vi "LangmuirProbeControlV2.vi"() -> ()   [LabVIEW 2014]
uses:
  <vilib>/express/express shared/transition.llb/Dynamic To Waveform Array.vi
  <vilib>/express/express arith-compare/Formula/Block/exnFormulaBlock how many pts in the wave.vi
  <vilib>/express/express shared/ex_Modify Signal Name.vi
  <vilib>/express/express shared/transition.llb/Waveform Array To Dynamic.vi
  <vilib>/express/express arith-compare/Formula/XNode/ExpressFormulaBlockNode.xnode
panel:
  in  "Min Voltage":dbl caption="Amplitude"
  in  "Max Voltage":dbl caption="Amplitude"
  in  "Log Data":bool
  out "I-V Curve":cluster{"Y":dbl[], "Y":dbl[]}[](graph)
  out "Waveform Graph":dynamicdata(graph)
  out "Resistor Voltage In":dbl
  out "Current Measure (V)":dynamicdata(graph) caption="data"
  out "Generated Signal":dynamicdata(graph) caption="Sine"
  in  "stop (F)":bool caption="STOP (F)"
  # "Desired Voltage Swing"
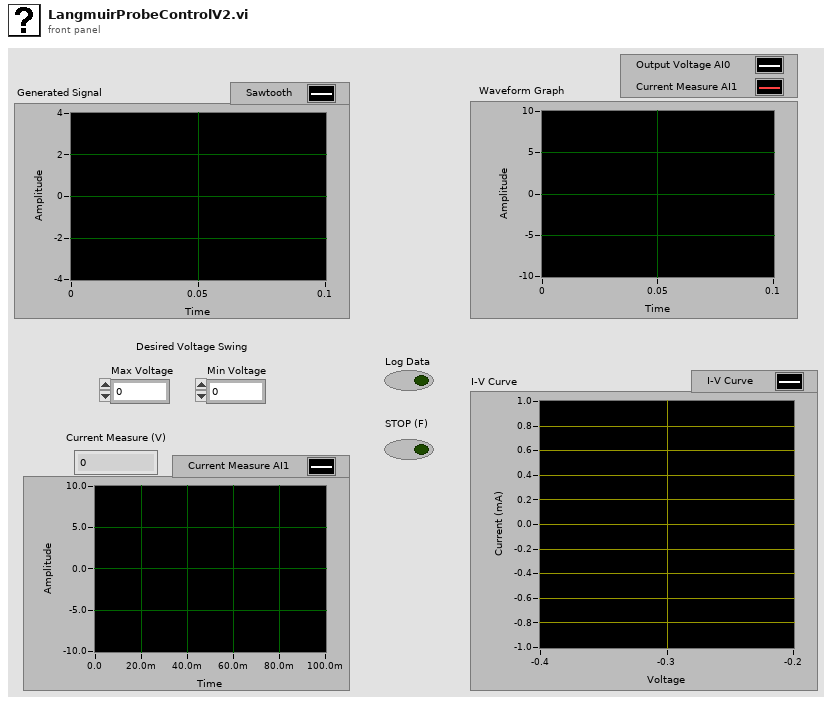
[diagram p1: front panel]
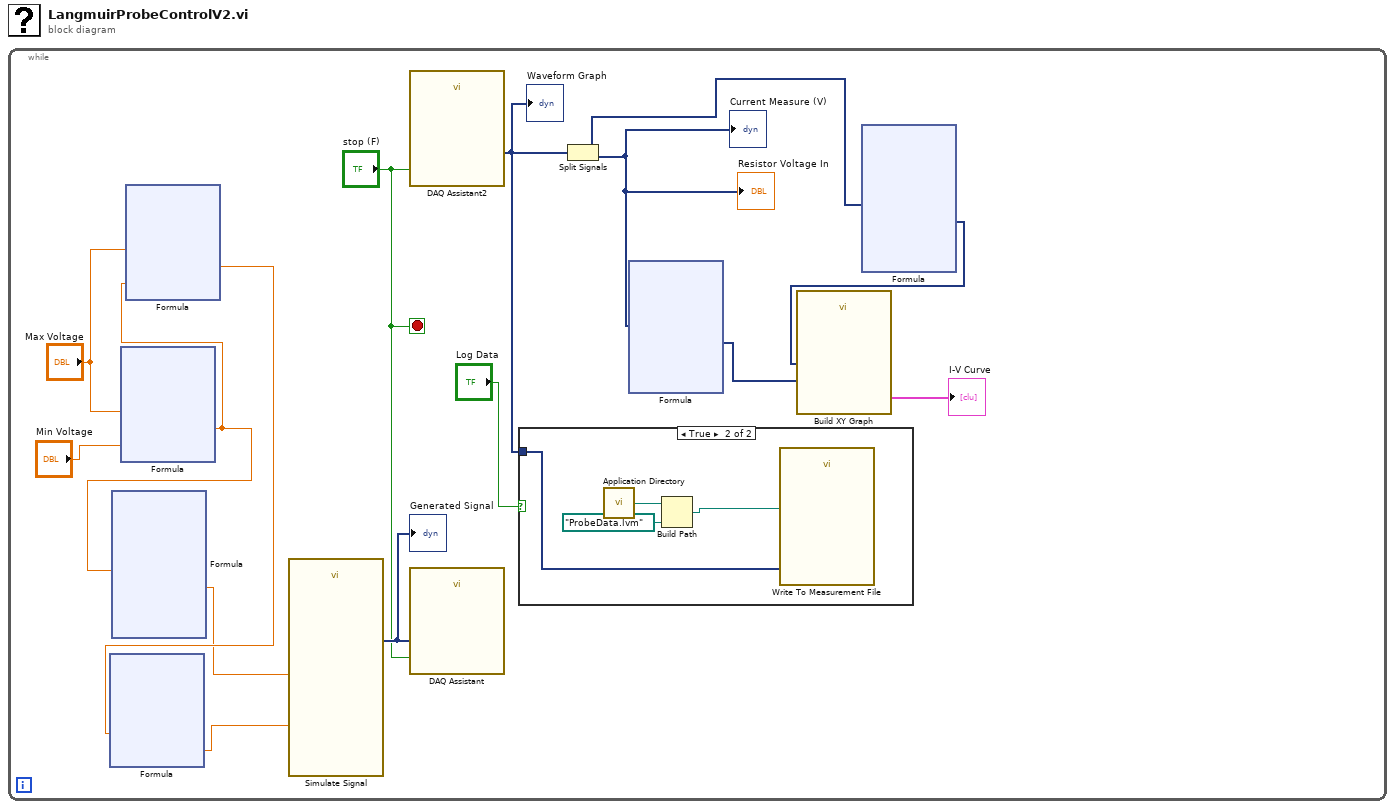
[diagram p0: block diagram]
diagram:
  n1 = while {
    stop <- "stop (F)" stop-if-true
    n2 = xnode "Formula"("X1"="Max Voltage", "X2"="Min Voltage") -> ("Result"=w6:dbl)  [unwired: 1 in, 1 out]
    n3 = xnode "Formula"("X1"=w6) -> ("Result"=w3:dbl)  [unwired: 1 in, 1 out]
    n4 = xnode "Formula"("X1"="Max Voltage", "X2"=w6) -> ("Result"=w5:dbl)  [unwired: 1 in, 1 out]
    n5 = xnode "Formula"("X1"=w5) -> ("Result"=w4:dbl)  [unwired: 1 in, 1 out]
    n6 = call "Simulate Signal"("Offset"=w4, "Amplitude"=w3) -> ("Sawtooth"=w14:dynamicdata)  [unwired: 12 in, 1 out]
    "Generated Signal" <- w14
    n7 = call "DAQ Assistant2"("stop (F)"="stop (F)") -> ("data"=w11:dynamicdata)  [unwired: 15 in, 3 out]
    "Waveform Graph" <- w11
    n8 = call "DAQ Assistant"("data"=w14, "stop (F)"="stop (F)") -> ()  [unwired: 15 in, 3 out]
    n9 = case shown="True" "Log Data" {
      tunnel: w11 -> [_ w194]
      frame False {
      }
      frame True {
        n10 = call <vilib>:"Application Directory.vi"() -> ("Application Directory"=w192:path)
        n11 = Build Path(base path=w192, name or relative path=path "ProbeData.lvm" ("ProbeData.lvm\nProbeData")) -> (appended path=w191:path)
        n12 = call "Write To Measurement File"("Signals"=w194, "Filename"=w191) -> ()  [unwired: 15 in, 3 out]
      }
    }
    n13 = Split Signals(w11) -> (w2:dynamicdata, w9:dynamicdata)  [unwired: 2 in]
    "Current Measure (V)" <- w9
    "Resistor Voltage In" <- w9
    n14 = xnode "Formula"("X1"=w9) -> ("Result"=w10:dynamicdata)  [unwired: 1 in, 1 out]
    n15 = xnode "Formula"("X1"=w2) -> ("Result"=w1:dynamicdata)  [unwired: 1 in, 1 out]
    n16 = call "Build XY Graph"("Y Input"=w10, "X Input"=w1) -> ("XY Graph"=→"I-V Curve":cluster{"X":dbl[], "Y":dbl[]}[])  [unwired: 8 in, 1 out]
  }
